vi "Sub_Connect_FGV.vi"(6 "timeout ms (20000)":i32=20000, 7 "MQTT Broker":cluster{"address (IP)":string, "port":u16}={"address (IP)"="broker.mqttdashboard.com", "port"=1883}, 8 "error in":errorcluster, 10 "Command":T1) -> (0 "error out":errorcluster, 3 "MQTT ref out":refnum<k5>)   [LabVIEW 2016, in "AWS_IoT.lvlib"]
uses:
  AWS_IoT.lvlib
  Controls/Conn_FGV_Cmds.ctl
  Controls/SSL_Connection.ctl
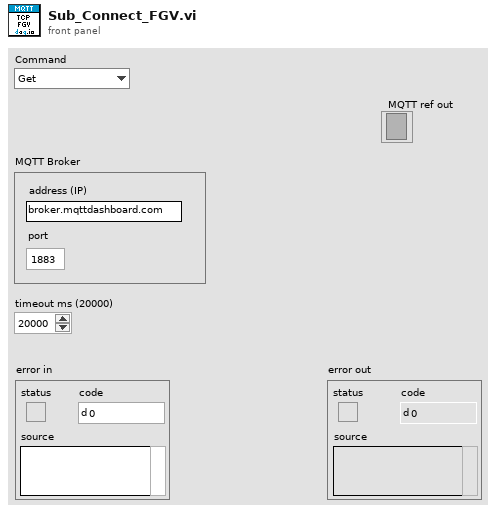
[diagram p1: front panel]
types:
  T1 = typedef "AWS_IoT.lvlib/Conn_FGV_Cmds.ctl" = enum16{"Get", "Set", "Delete"}
  T2 = typedef "AWS_IoT.lvlib/SSL_Connection.ctl" = cluster{"connection ID":refnum<k5>, "TLS":cluster{"CXT ptr":i32, "SSL ptr":i32, "Socket ptr":i32}, "NIssleay library path":path, "server url":string}
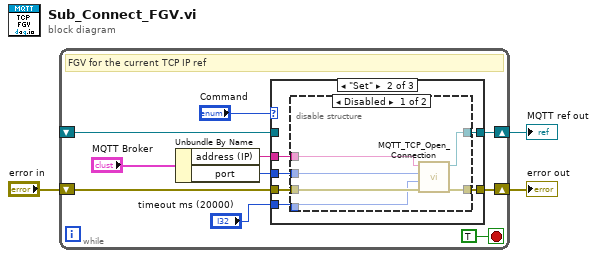
[diagram p0: block diagram]
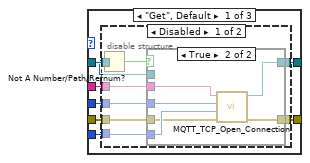
[diagram p2: hidden frame]
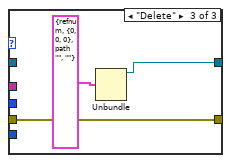
[diagram p6: hidden frame]
diagram:
  n1 = while {
    shift-right: [w7] -> w1
    shift-left: "error in" -> [w8]
    shift-right: [w6] -> w3
    shift-left: _ -> [w5]
    stop <- TRUE stop-if-true
    # "FGV for the current TCP IP ref"
    n2 = Unbundle By Name("MQTT Broker") -> ("address (IP)"=w10:string, "port"=w9:u16)
    n3 = case shown="\"Set\"" "Command" {
      tunnel: w10 -> [w20 w42 _]
      tunnel: w9 -> [w19 w41 _]
      tunnel: w8 -> [w17 w40 w51]
      tunnel: [w16 w39 w51] -> w7
      tunnel: [w15 w38 w49] -> w6
      tunnel: w5 -> [w14 _ _]
      tunnel: "timeout ms (20000)" -> [w18 w37 _]
      frame "Get", Default {
        n4 = disable-structure shown="Disabled" {
          disable-tunnel: w20 -> [w27 _]
          disable-tunnel: w19 -> [w26 _]
          disable-tunnel: w18 -> [w25 _]
          disable-tunnel: w17 -> [w24 _]
          disable-tunnel: [w23 _] -> w16
          disable-tunnel: [w22 _] -> w15
          disable-tunnel: w14 -> [w21 _]
          frame Disabled {
            n5 = Not A Number/Path/Refnum?(number/path/refnum=w21) -> (NaN/Path/Refnum?=w28:bool)
            n6 = case shown="True" w28 {
              tunnel: w27 -> [_ w36]
              tunnel: w26 -> [_ w35]
              tunnel: w25 -> [_ w34]
              tunnel: w24 -> [w29 w33]
              tunnel: [w29 w32] -> w23
              tunnel: [w30 w31] -> w22
              tunnel: w21 -> [w30 _]
              frame False {
                # "existing refnum\nis likely good"
              }
              frame True {
                n7 = call "MQTT_TCP_Open_Connection.vi"("error in (no error)"=w33, "timeout ms (20000)"=w34, "remote port or service name"=w35, "address"=w36) -> ("error out"=w32:errorcluster, "connection ID"=w31:refnum<k5>)  [unwired: 6 in]
              }
            }
          }
          frame Enabled {
          }
        }
      }
      frame "Set" {
        n8 = disable-structure shown="Disabled" {
          disable-tunnel: w42 -> [w48 _]
          disable-tunnel: w41 -> [w47 _]
          disable-tunnel: w40 -> [w46 _]
          disable-tunnel: [w45 _] -> w39
          disable-tunnel: [w44 _] -> w38
          disable-tunnel: w37 -> [w43 _]
          frame Disabled {
            n9 = call "MQTT_TCP_Open_Connection.vi"("error in (no error)"=w46, "timeout ms (20000)"=w43, "remote port or service name"=w47, "address"=w48) -> ("error out"=w45:errorcluster, "connection ID"=w44:refnum<k5>)  [unwired: 6 in]
          }
          frame Enabled {
          }
        }
      }
      frame "Delete" {
        n10 = Unbundle(T2 {"connection ID"=refnum, "TLS"={"CXT ptr"=0, "SSL ptr"=0, "Socket ptr"=0}, "NIssleay library path"=path "", "server url"=""} ("SSL_Connection")) -> ("connection ID"=w49:refnum<k5>)  [unwired: 3 out]
      }
    }
  }
  "MQTT ref out" <- w3
  "error out" <- w1
